vi "simple_publisher.vi"() -> ()   [LabVIEW 2014]
panel:
  in  "停止":bool
  out "JSON字符串":string
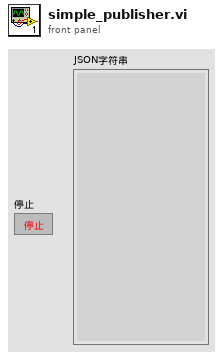
[diagram p1: front panel]
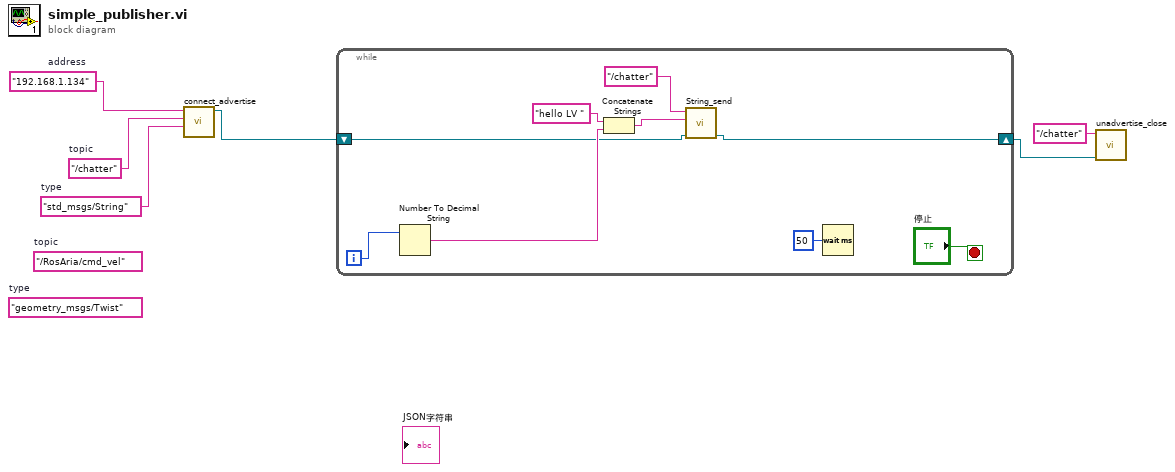
[diagram p0: block diagram]
diagram:
  w6 = "192.168.1.134"  # address
  w4 = "std_msgs/String"  # type
  w5 = "/chatter"  # topic
  (unwired) "geometry_msgs/Twist"  # type
  (unwired) "/RosAria/cmd_vel"  # topic
  n1 = call "connect_advertise.vi"("type"=w4, "topic"=w5, "address"=w6) -> ("连接ID输出"=w3:refnum<k5>)  [unwired: 7 in, 1 out]
  n2 = while {
    shift-right: [w7] -> w2
    shift-left: w3 -> [w8]
    i -> [w11]
    stop <- "停止" stop-if-true
    n3 = Number To Decimal String(number=w11) -> (decimal integer string=w10:string)  [unwired: 1 in]
    n4 = Concatenate Strings("hello LV " ("data"), w10) -> (w9:string)
    n5 = call "String_send.vi"("连接ID"=w8, "data"=w9, "topic"="/chatter") -> ("连接ID输出"=w7:refnum<k5>)  [unwired: 7 in, 1 out]
    n6 = Wait (ms)(milliseconds to wait=u32 50 ("等待时间（毫秒）")) -> ()  [unwired: 1 out]
  }
  n7 = call "unadvertise_close.vi"("连接ID"=w2, "topic"="/chatter") -> ()  [unwired: 10 in]
